vi "2283_controlDePistones.vi"(0 "Boton 1":bool, 5 "Boton 2":bool) -> (1 "solenoideCuernito":T1, 4 "solenoideGarra":T1, 7 "Motor":dbl)   [LabVIEW 2014]
uses:
  <vilib>/Rock Robotics/WPI/Solenoid/WPI_SolenoidValue.ctl
panel:
  in  "Output":dbl format="%#_13g"
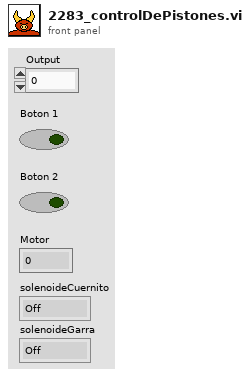
[diagram p1: front panel]
types:
  T1 = typedef "WPI_SolenoidValue.ctl" = enum16{"Off", "On", "Forward", "Reverse"}
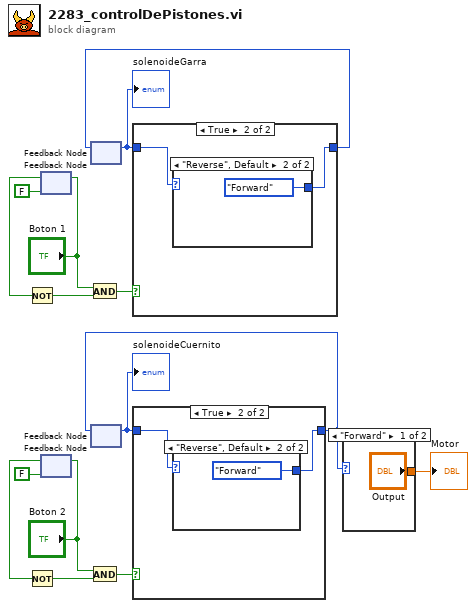
[diagram p0: block diagram]
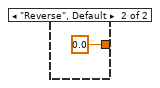
[diagram p2: hidden frame]
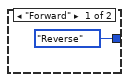
[diagram p4: hidden frame]
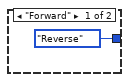
[diagram p6: hidden frame]
diagram:
  n1 = feedback #1(FALSE) -> (w10:bool)
  n2 = Not(x=w10) -> (.not. x?=w9:bool)
  n3 = feedback-in #1("Boton 1") -> ()
  n4 = feedback #2(FALSE) -> (w14:bool)
  n5 = Not(x=w14) -> (.not. x?=w13:bool)
  n6 = feedback-in #2("Boton 2") -> ()
  n7 = And(x="Boton 1", y=w9) -> (x .and. y?=w8:bool)
  n8 = And(x="Boton 2", y=w13) -> (x .and. y?=w12:bool)
  n9 = feedback #3() -> (w6:T1)  [unwired: 1 in]
  "solenoideGarra" <- w6
  n10 = feedback #4() -> (w1:T1)  [unwired: 1 in]
  "solenoideCuernito" <- w1
  n11 = case shown="True" w8 {
    tunnel: [w16 w18] -> w7
    tunnel: w6 -> [w16 w17]
    frame False {
    }
    frame True {
      n12 = case shown="\"Reverse\", Default" w17 {
        tunnel: [WPI_SolenoidValue."Reverse" ("Value") WPI_SolenoidValue."Forward" ("Value")] -> w18
        frame "Forward" {
        }
        frame "Reverse", Default {
        }
      }
    }
  }
  n13 = feedback-in #3(w7) -> ()
  n14 = case shown="True" w12 {
    tunnel: [w21 w23] -> w5
    tunnel: w1 -> [w21 w22]
    frame False {
    }
    frame True {
      n15 = case shown="\"Reverse\", Default" w22 {
        tunnel: [WPI_SolenoidValue."Reverse" ("Value") WPI_SolenoidValue."Forward" ("Value")] -> w23
        frame "Forward" {
        }
        frame "Reverse", Default {
        }
      }
    }
  }
  n16 = feedback-in #4(w5) -> ()
  n17 = case shown="\"Forward\"" w5 {
    tunnel: ["Output" 0.0 ("Output")] -> w2
    frame "Forward" {
    }
    frame "Reverse", Default {
    }
  }
  "Motor" <- w2
